vi "ziCheckVersion.vi"(0 "Handle In":T1 {"Handle" format="0x%08x"; "Conn" format="0x%08x"}, 11 "Error In":errorcluster) -> (4 "Handle Out":T1 {"Handle" format="0x%08x"; "Conn" format="0x%08x"}, 8 "Message":string, 15 "Error Out":errorcluster)   [LabVIEW 2019, in "Zurich Instruments LabOne.lvlib"]
doc: "Checks if Version of API and DataServer are the same and reports a user dialog with warning if not."
uses:
  <instrlib>/Zurich Instruments LabOne/Zurich Instruments LabOne.lvlib
  <instrlib>/Zurich Instruments LabOne/Public/ziTypeHandle.ctl
  <instrlib>/Zurich Instruments LabOne/Public/Configure/ziGetValueString.vi
  <instrlib>/Zurich Instruments LabOne/Public/Configure/ziGetValueDouble.vi
  <instrlib>/Zurich Instruments LabOne/Private/ziLV64.dll
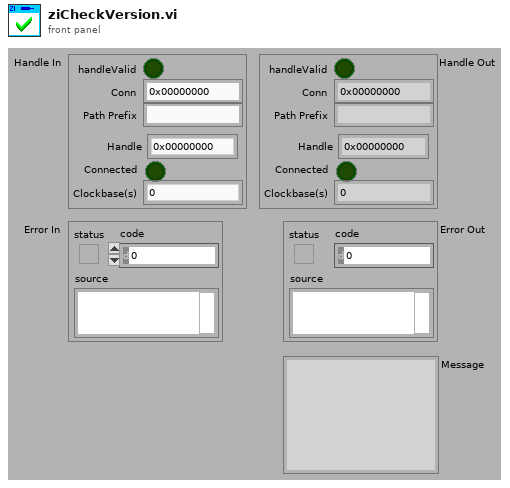
[diagram p1: front panel]
types:
  T1 = typedef "Zurich Instruments LabOne.lvlib/ziTypeHandle.ctl" = cluster{"handleValid":bool, "Conn":u64, "Path Prefix":string, "Handle":u64, "Connected":bool, "Clockbase(s)":dbl}
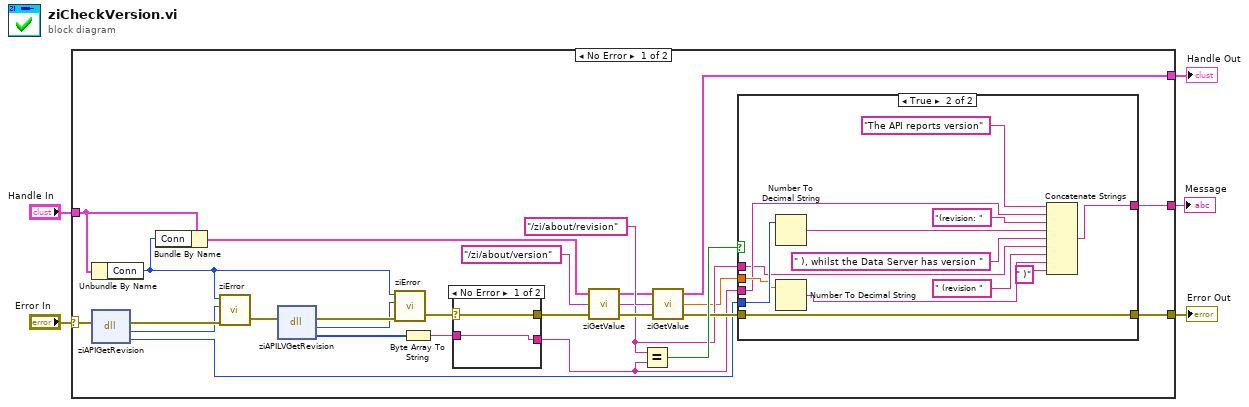
[diagram p0: block diagram]
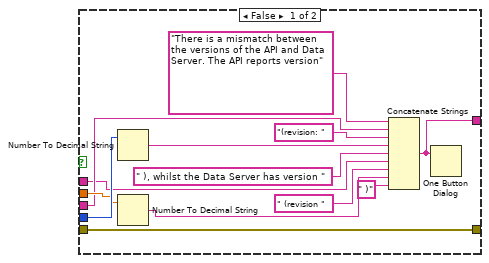
[diagram p2: hidden frame]
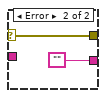
[diagram p3: hidden frame]
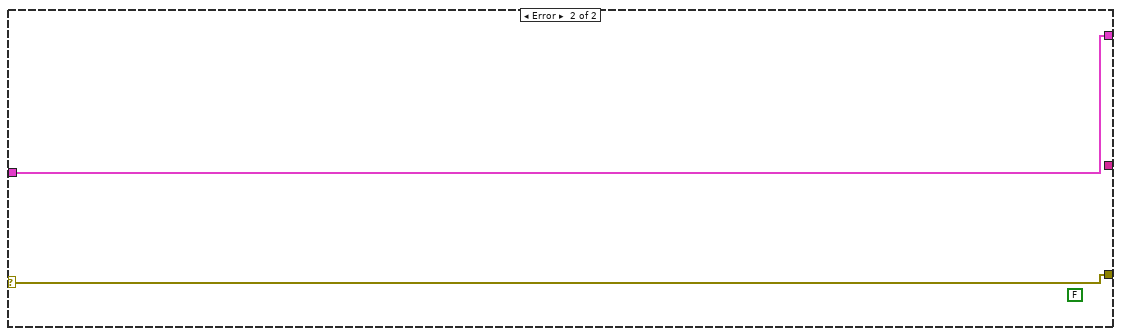
[diagram p4: hidden frame]
diagram:
  n1 = case shown="No Error" "Error In" {
    selector: "Error In" -> [w18 w63]
    tunnel: [w26 w63] -> w5
    tunnel: [w20 w62] -> w4
    tunnel: "Handle In" -> [w30 w62]
    tunnel: [w6 _] -> w1
    frame No Error {
      n2 = Unbundle By Name(w30) -> ("Conn"=w7:u64)
      n3 = dll-call lib="C:/Program Files/National Instruments/LabVIEW 2019/instr.lib/Zurich Instruments LabOne/Private/ziLV*.*" fn="ziAPIGetRevision"(error in=w18) -> (error out=w19:errorcluster, "return type"=w17:u32, "revision"=w13:u32)  [unwired: 2 in, 2 out]
      n4 = Bundle By Name(cluster=w30, "Conn"=w7) -> (w29:T1)
      n5 = call <instrlib>:"ziError.vi"("Conn"=w7, "ziErrorCode"=w17, "Error In"=w19) -> ("Error Out"=w10:errorcluster)  [unwired: 3 in]
      n6 = dll-call lib="C:/Program Files/National Instruments/LabVIEW 2019/instr.lib/Zurich Instruments LabOne/Private/ziLV*.*" fn="ziAPILVGetRevision"(error in=w10) -> (error out=w9:errorcluster, "return type"=w8:u32, "Conn"=w11:u8[])  [unwired: 3 in, 1 out]
      n7 = call <instrlib>:"ziError.vi"("Conn"=w7, "ziErrorCode"=w8, "Error In"=w9) -> ("Error Out"=w31:errorcluster)  [unwired: 3 in]
      n8 = Byte Array To String(unsigned byte array=w11) -> (string=w12:string)
      n9 = case shown="No Error" w31 {
        selector: w31 -> [w59 w61]
        tunnel: [w59 w61] -> w28
        tunnel: w12 -> [w58 _]
        tunnel: [w58 ""] -> w15
        frame No Error {
        }
        frame Error {
        }
      }
      n10 = call-poly <instrlib>:"ziGetValue.vi"("error in"=w28, "Path"="/zi/about/version", "Handle In"=w29) -> ("error out"=w22:errorcluster, "Value"=w16:string, "Handle Out"=w23:T1)
      n11 = Equal?(x=w16, y=w15) -> (x = y?=w27:bool)
      n12 = call-poly <instrlib>:"ziGetValue.vi"("error in"=w22, "Path"="/zi/about/revision", "Handle in"=w23) -> ("error out"=w21:errorcluster, "Value"=w14:dbl, "Handle out"=w20:T1)
      n13 = case shown="True" w27 {
        tunnel: w21 -> [w37 w50]
        tunnel: [w37 w50] -> w26
        tunnel: w16 -> [w33 w46]
        tunnel: w15 -> [w34 w47]
        tunnel: w14 -> [w35 w48]
        tunnel: w13 -> [w36 w49]
        tunnel: [w32 w45] -> w6
        frame False {
          n14 = Number To Decimal String(number=w36) -> (decimal integer string=w40:string)  [unwired: 1 in]
          n15 = Number To Decimal String(number=w35) -> (decimal integer string=w39:string)  [unwired: 1 in]
          n16 = Concatenate Strings("There is a mismatch between the versions of the API and Data Server. The API reports version" ("[error source] (\" \")"), w34, "(revision: " ("[error source] (\" \")"), w40, " ), whilst the Data Server has version " ("[error source] (\" \")"), w33, " (revision " ("[error source] (\" \")"), w39, " )" ("[error source] (\" \")")) -> (w32:string)
          n17 = One Button Dialog(message=w32) -> ()  [unwired: 1 in, 1 out]
        }
        frame True {
          n18 = Number To Decimal String(number=w49) -> (decimal integer string=w53:string)  [unwired: 1 in]
          n19 = Number To Decimal String(number=w48) -> (decimal integer string=w52:string)  [unwired: 1 in]
          n20 = Concatenate Strings("The API reports version" ("[error source] (\" \")"), w47, "(revision: " ("[error source] (\" \")"), w53, " ), whilst the Data Server has version " ("[error source] (\" \")"), w46, " (revision " ("[error source] (\" \")"), w52, " )" ("[error source] (\" \")")) -> (w45:string)
        }
      }
    }
    frame Error {
      (unwired) FALSE
    }
  }
  "Error Out" <- w5
  "Handle Out" <- w4
  "Message" <- w1
